vi "时间坐标.vi"() -> ()   [LabVIEW 2022 SP3]
doc: "本VI是为《我和LabVIEW》一书编写的示例。\n关于本书的介绍请参考网页：\nhttp://ruanqizhen.spaces.live.com/blog/cns!5852D4F797C53FB6!4310.entry"
panel:
  out "波形数据":waveform(dbl) caption="波形输出"
  out "波形曲线":waveform(dbl)(graph) caption="(Y) Single Plot"
  # "Instructions:\nRun the VI and investigate the different types of graphs."
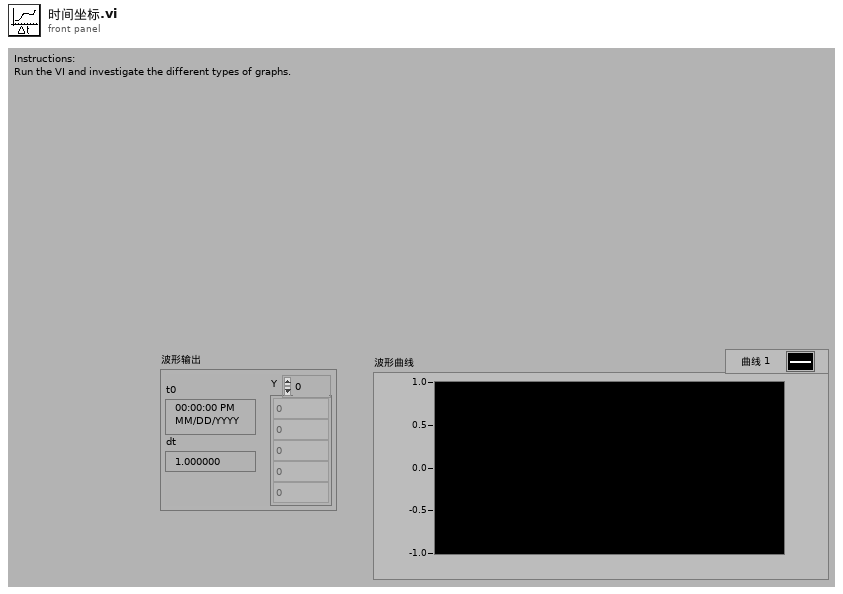
[diagram p1: front panel]
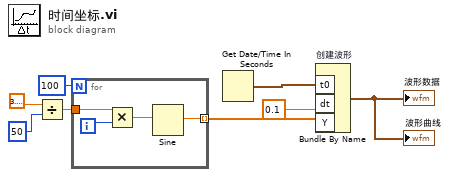
[diagram p0: block diagram]
diagram:
  n1 = Divide(x=3.141592653589793, y=50) -> (x/y=w7:dbl)
  n2 = for {
    N: 100 -> [_]
    tunnel: w7 -> [w12]
    tunnel: [w9] -> w4 mode=indexing
    i -> [w11]
    n3 = Multiply(x=w12, y=w11) -> (x*y=w10:dbl)
    n4 = Sine(x=w10) -> (sin(x)=w9:dbl)
  }
  n5 = Get Date/Time In Seconds() -> (seconds since 1Jan1904=w2:timestamp)
  n6 = Bundle By Name "创建波形"("t0"=w2, "dt"=0.1, "Y"=w4) -> (→"波形曲线" →"波形数据":waveform(dbl))  [unwired: 1 out]
